vi "PH_PILS.destructor.vi"(0 "i ref in":refnum<vi>, 5 "error in(no error)":errorcluster) -> (19 "error out":errorcluster)   [LabVIEW 2014, in "PH_PILS.lvlib"]
doc: "This is the destructor of a class.\n\nLicense Agreement for this software:\n\nCopyright (C)\nGesellschaft für Schwerionenforschung, GSI\nPlanckstr. 1\n64291 Darmstadt\nGermany\n\nContact: D.Beck@gsi.de \n\nThis program is free software; you can redistribute it and/or modify it under the terms of the \nGNU General Public License as published by the Free Software Foundation; either version 2 of \nthe license, or (at your option) any later version.\n\nThis program is distributed in the hope that it will be useful, but WITHOUT ANY WARRANTY; \nwithout even the implied warranty of MERCHANTABILITY or FITNESS FOR A PARTICULAR PURPOSE. See the GNU General License for more details (http://www.gnu.org).\n\nGesellschaft für Schwerionenforschung, GSI\nPlanckstr. 1, 64291 Darmstadt, Germany\nFor all questions and ideas contact: M.Richter@gsi.de, H.Brand@gsi.de or D.Beck@gsi.de.\nLast update: 16-JUN-2004"
uses:
  PH_PILS.lvlib
  PH_Basics/PH_SystemInformation/PH_SystemInformation.lvlib
  PH_Devices/PH_Beckhoff/PH_Beckhoff.lvlib
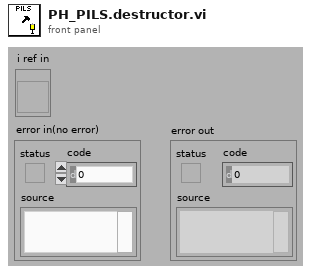
[diagram p1: front panel]
types:
  T1 = enum16{"SetAttribute", "GetAttribute", "CreateAttribute", "DestroyAttribute", "DestroyAllAtributes"}
  T2 = typedef "PH_PILS.lvlib/PH_PILS.i attribute.ctl" = cluster{"Boolean":cluster{"GUI Ref":refnum<vi>, "Status":i32}[], "GUI Refs Exp. Shutters":cluster{"1":refnum<vi>, "2":refnum<vi>, "3":refnum<vi>, "4":refnum<vi>}, "Tristate2Run GUI Refs":refnum<vi>[], "EO-Likes":cluster{"GUI Ref":refnum<vi>, "Status":i32}[], "Operation Mode":cluster{"Operation Mode":T3, "GUI":cluster{"Ref State":refnum<vi>, "Ref":refnum<vi>}, "Servicemode":cluster{"Tagname":string, "Status":i32}, "Labormode":cluster{"Tagname":string, "Status":i32}, "Searchmode":cluster{"Tagname":string, "Status":i32}, "Shotmode":cluster{"Tagname":string, "Status":i32}}, "Submode":cluster{"Submode":T4, "GUI":cluster{"Ref State":refnum<vi>, "Ref":refnum<vi>}, "Submode":cluster{"Tagname":string, "Status":i32}}, "Experiment":cluster{"Experiment":enum16{"unknown", "intern", "4 (Z6)", "3", "2", "1"}, "GUI":cluster{"Ref State":refnum<vi>, "Ref":refnum<vi>}, "intern":cluster{"Tagname":string, "Status":i32}, "Exp 4":cluster{"Tagname":string, "Status":i32}, "Exp 3":cluster{"Tagname":string, "Status":i32}, "Exp 2":cluster{"Tagname":string, "Status":i32}, "Exp 1":cluster{"Tagname":string, "Status":i32}}, "TristateNormal":cluster{"GUI Ref":refnum<vi>, "Status":i32}[], "Door Tags":cluster{"GUI Ref":refnum<vi>, "Status":i32}[], "GUIlessTags":cluster{"Name":string, "Status":i32}[], "Beamline GUI Refs":refnum<vi>[], "Special Boolean":cluster{"GUI Ref":refnum<vi>, "Status":i32}[], "Laserpower":cluster{"GUI Ref":refnum<vi>, "Status":i32}[], "Shutter":cluster{"GUI Ref":refnum<vi>, "Status":i32}[], "Tristate EO Like":cluster{"GUI Ref":refnum<vi>, "Status":i32}[], "PP":cluster{"GUI Ref":refnum<vi>, "Status":i32, "Head Ref":refnum<vi>, "Slider Ref":refnum<vi>}[], "Switch Knobs":cluster{"GUI Ref":refnum<vi>, "Status":i32}[], "Latch Knob GUI Refs":refnum<vi>[], "FailureCounter":i32, "Enabled Status":cluster{"Laser":i32, "PreAmp":i32, "MainAmp":i32}, "Mercury":refnum<vi>, "Instance Rods":string, "Logfile":path, "Beckhoff-Instance Internal":string, "Beckhoff-Instance External":string, "Enabling Rights":cluster{"Name":string, "Password":string, "PA?":bool, "MA?":bool, "Exp?":bool}[]}
  T3 = typedef "PH_PILS.lvlib/PH_PILS.Operation Mode.ctl" = enum16{"unknown", "Service", "Labor", "Search", "Shot"}
  T4 = typedef "PH_PILS.lvlib/PH_PILS.Submode.ctl" = enum16{"unknown", "HV-Normal", "HV-Test"}
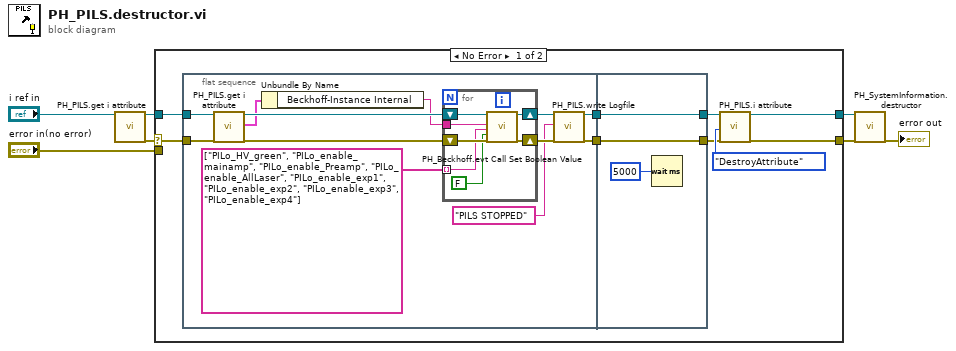
[diagram p0: block diagram]
diagram:
  n1 = call "PH_PILS.get i attribute.vi"("i ref in"="i ref in") -> ("i ref out"=w5:refnum<vi>, "error out"=w4:errorcluster)  [unwired: 16 in, 1 out]
  n2 = case shown="No Error" w4 {
    selector: w4 -> [w8 _]
    tunnel: [w11 w39] -> w7
    tunnel: [w10 w40] -> w2
    tunnel: w5 -> [w9 w40]
    tunnel: "error in(no error)" -> [_ w39]
    frame No Error {
      n3 = flat-sequence {
        tunnel: w9 -> [w28]
        tunnel: w8 -> [w27]
        tunnel: [w20] -> w16
        tunnel: [w18] -> w15
        tunnel: [w37] -> w12
        tunnel: [w38] -> w13
        tunnel: w16 -> [w38]
        tunnel: w15 -> [w37]
        frame #0 {
          n4 = call "PH_PILS.get i attribute.vi"("i ref in"=w28, "error in (no error)"=w27) -> ("i ref out"=w25:refnum<vi>, "i attribute"=w23:T2, "error out"=w26:errorcluster)  [unwired: 15 in]
          n5 = Unbundle By Name(w23) -> ("Beckhoff-Instance Internal"=w22:string)
          n6 = for {
            tunnel: w22 -> [w33]
            tunnel: string[] ["PILo_HV_green", "PILo_enable_mainamp", "PILo_enable_Preamp", "PILo_enable_AllLaser", "PILo_enable_exp1", "PILo_enable_exp2", "PILo_enable_exp3", "PILo_enable_exp4"] -> [w30] mode=indexing
            shift-right: [w35] -> w21
            shift-left: w26 -> [w34]
            shift-right: [w31] -> w19
            shift-left: w25 -> [w32]
            n7 = call "PH_Beckhoff.evt Call Set Boolean Value.vi"("i ref in"=w32, "Beckhoff Instance"=w33, "Tagname to set"=w30, "Value"=FALSE ("Value to set"), "error in"=w34) -> ("i ref out"=w31:refnum<vi>, "error out"=w35:errorcluster)  [unwired: 13 in]
          }
          n8 = call "PH_PILS.write Logfile.vi"("i ref in"=w19, "Text"="PILS STOPPED" ("string"), "error in"=w21) -> ("i ref out"=w18:refnum<vi>, "error out"=w20:errorcluster)  [unwired: 15 in]
        }
        frame #1 {
          n9 = Wait (ms)(milliseconds to wait=u32 5000) -> ()  [unwired: 1 out]
        }
      }
      n10 = call "PH_PILS.i attribute.vi"("VI Refnum"=w12, "Action"=T1."DestroyAttribute", "error in (no error)"=w13) -> ("VI Refnum out"=w10:refnum<vi>, "error out"=w11:errorcluster)  [unwired: 14 in, 1 out]
    }
    frame Error {
    }
  }
  n11 = call "PH_SystemInformation.destructor.vi"("i ref in"=w2, "error in(no error)"=w7) -> ("error out"=→"error out":errorcluster)  [unwired: 17 in]
